vi "ni579x Host Align.vi"(0 "sync.resources":T1, 1 "sync.meas.Reference Clock":refnum<k21>, 2 "sync.meas.FPGA Clock x2":refnum<k21>, 3 "sync.meas.FPGA I/O":refnum<k21>) -> (4 "sync.resources":T1)   [LabVIEW 2013, in "ni579x Synchronization v1 FPGA.lvlib"]
doc: "*** THIS VI IS DEPRECATED. USE ni579x Host Align 2.vi ***\n\nAlign the targets participating in synchronization. This must occur before a signal can be synchronized.\n\nThere are two flavors of alignment to chose from -- Host Align and FPGA Align. The two flavors produce the same quality of synchronization, but differ in requirements and versatility of operation.\n\nWhen using <B>ni579x FPGA Align 2</B>, the Single Cycle Timed Loop (SCTL) rate (that this VI is in) must be an integer multiple of the <B>sync.cptr.Reference Clock</B> rate, and the SCTL clock must have a fixed phase relationship to the reference clock. Each target performs its alignment independently, so FPGA Align does not require a FPGA I/O line. It's also possible to use FPGA Align without host interaction. FPGA Align has 100% repeatability if-and-only-if the target-to-target phase relationship is low and does not change.\n\nWhen using <B>ni579x Host Align 2</B>, the SCTL rate may be arbitrary (yet still must have a fixed phase relationship to the other targets). The CPTR period may also be arbitrary. This alignment process is coordinated by the host, and requires an FPGA I/O line for orchestration. Host Align has 100% repeatability; if the hardware configuration remains constant, so will the level of synchronization.\n\n<B>Input Parameters</B>\n\n<B>sync.resources</B> identifies the Synchronization instance. 'sync.resources' is obtained from the ni579x Create VI of this library.\n\n<B>sync.meas.Reference Clock</B> is used by the measurement logic as the \"start\" signal. This is commonly PXI_Clk10.\n\n<B>sync.meas.FPGA Clock x2</B> is used by the measurement logic as the measurement clock. This clock must run at twice the rate of the FPGA Clock (the clock that drives the Single Cycle Timed Loop (SCTL) which this VI is in). This clock must also be derrived from the FPGA Clock, so that it has a fixed phase relationship. This is commonly IO Module\\Sample Clock x2.\n\n<B>sync.meas.FPGA I/O</B> is the FPGA I/O line that will be used to orchestrate starting the measurements. This is commonly a PXI Trig line.\n\nNote: For large NI chassis, make sure the PXI Trig line is routed to all bus segments that have targets participating in synchronization.\n\n<B>Output Parameters</B>\n\n<B>sync.resources</B> is the same instance that was passed in for 'sync.resources'."
uses:
  <instrlib>/ni579x/Synchronization/v1/FPGA/ni579x Synchronization v1 FPGA.lvlib
  <instrlib>/ni579x/Synchronization/v1/FPGA/Implementation/Resources.ctl
  <vilib>/rvi/eio/common/nirviEmuReportErrorAndStop.vi
  <vilib>/rvi/DataTransferAndStorage/Container/Common/niFpgaContainerSetEmuInfo.vi
  <vilib>/rvi/DataTransferAndStorage/Container/Common/niFpgaContainerGetUniqueNameForEmu.vi
  <vilib>/rvi/eio/common/nirviEmuTemplateMethod_errors.vi
  <vilib>/rvi/LocalResourceManager/LocalResourceManager.xnode
  <vilib>/eio/EIONode/EIONode.xnode
  <instrlib>/_niInstr/Basic Elements/v1/FPGA/niInstr Basic Elements v1 FPGA.lvlib
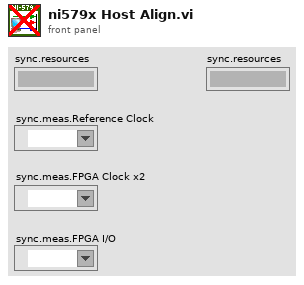
[diagram p1: front panel]
types:
  T1 = typedef "ni579x Synchronization v1 FPGA.lvlib/Resources.ctl" = cluster{"master":refnum<k21>, "meas.enable":refnum<k21>, "meas.ready":refnum<k21>, "meas.arm":refnum<k21>, "meas.valid":refnum<k21>, "meas.value":refnum<k21>, "meas.oversample clock":refnum<k21>, "meas.oversample factor":refnum<k21>, "cptr":refnum<k21>, "cptr.adjust":refnum<k21>, "cptr.period":refnum<k21>}
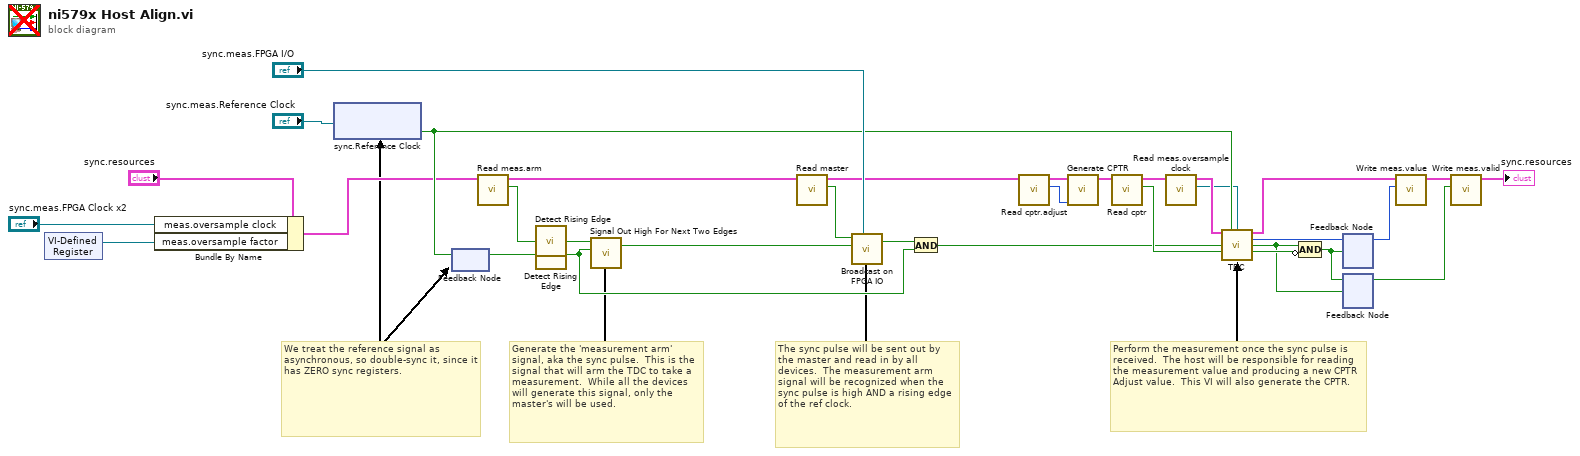
[diagram p0: block diagram]
diagram:
  # "We treat the reference signal as asynchronous, so double-sync it, since it has ZERO sync registers."
  # "Perform the measurement once the sync pulse is received.  The host will be responsible for reading the measurement value and producing a new CPTR Adjust value.  This VI will also generate the CPTR."
  # "The sync pulse will be sent out by the master and read in by all devices.  The measurement arm signal will be recognized when the sync pulse is high AND a rising edge of the ref clock."
  # "Generate the 'measurement arm' signal, aka the sync pulse.  This is the signal that will arm the TDC to take a measurement.  While all the devices will generate this signal, only the master's will be used."
  n1 = xnode "VI-Defined Register"() -> ("Register Out"=w4:refnum<k21>)
  n2 = Bundle By Name(cluster="sync.resources", "meas.oversample clock"="sync.meas.FPGA Clock x2", "meas.oversample factor"=w4) -> (w2:T1)
  n3 = xnode ("sync.Reference Clock")("FPGA I/O In"="sync.meas.Reference Clock") -> ("I/O Item"=w23:bool)  [unwired: 1 out]
  n4 = feedback #1() -> (w30:bool)  [unwired: 1 in]
  n5 = feedback-in #1(w23) -> ()
  n6 = call <instrlib>:"Read meas.arm.vi"("sync.resources"=w2) -> ("meas.arm"=w26:bool, "sync.resources"=w18:T1)  [unwired: 9 in]
  n7 = call <instrlib>:"Detect Rising Edge.vi"("signal"=w26) -> ("edge detected"=w31:bool)  [unwired: 14 in]
  n8 = call <instrlib>:"Detect Rising Edge.vi"("signal"=w30) -> ("edge detected"=w33:bool)  [unwired: 14 in]
  n9 = call <instrlib>:"Signal Out High For Next Two Edges.vi"("edge"=w33, "signal"=w31) -> ("signal for distribution"=w29:bool)  [unwired: 3 in]
  n10 = call <instrlib>:"Read master.vi"("sync.resources"=w18) -> ("master"=w25:bool, "sync.resources"=w13:T1)  [unwired: 9 in]
  n11 = call <instrlib>:"Broadcast on FPGA IO.vi"("FPGA I/O"="sync.meas.FPGA I/O", "signal in"=w29, "master"=w25) -> ("signal out"=w28:bool)  [unwired: 4 in]
  n12 = And(x=w28, y=w33) -> (x .and. y?=w1:bool)
  n13 = call <instrlib>:"Read cptr.adjust.vi"("sync.resources"=w13) -> ("cptr.adjust"=w12:u16, "sync.resources"=w14:T1)  [unwired: 9 in]
  n14 = call <instrlib>:"Generate CPTR.vi"("sync.cptr.adjust"=w12, "sync.resources"=w14) -> ("sync.resources"=w11:T1)  [unwired: 9 in]
  n15 = call <instrlib>:"Read cptr.vi"("sync.resources"=w11) -> ("cptr"=w24:bool, "sync.resources"=w9:T1)  [unwired: 9 in]
  n16 = call <instrlib>:"Read meas.oversample clock.vi"("sync.resources"=w9) -> ("meas.oversample clock"=w6:refnum<k21>, "sync.resources"=w7:T1)  [unwired: 9 in]
  n17 = call <instrlib>:"TDC.vi"("sync.resources"=w7, "sync.Reference Clock"=w23, "sync.meas.oversample clock"=w6, "sync.meas.arm"=w1, "sync.cptr"=w24) -> ("sync.resources"=w8:T1, "count out"=w21:u16, "count valid"=w15:bool, "rollover error"=w16:bool)  [unwired: 6 in, 1 out]
  n18 = Compound Arithmetic op=AND(w15, invert w16) -> (w22:bool)
  n19 = feedback #2() -> (w20:u16)  [unwired: 1 in]
  n20 = feedback-in #2(w21, w22) -> ()
  n21 = feedback #3() -> (w19:bool)  [unwired: 1 in]
  n22 = feedback-in #3(w22, w15) -> ()
  n23 = call <instrlib>:"Write meas.value.vi"("meas.value"=w20, "sync.resources"=w8) -> ("sync.resources"=w17:T1)  [unwired: 9 in]
  n24 = call <instrlib>:"Write meas.valid.vi"("meas.valid"=w19, "sync.resources"=w17) -> ("sync.resources"=→"sync.resources":T1)  [unwired: 9 in]
